vi "SetMenuDisplayed.vi"(8 "error in (no error)":errorcluster, 9 "Displayed":bool, 10 "Tag":string, 11 "Menu in":refnum<class "Menu.lvclass">) -> (0 "error out":errorcluster, 3 "Menu out":refnum<class "Menu.lvclass">)   [LabVIEW 2021, in "Menu.lvlib" / "Menu.lvclass"]
uses:
  Menu.lvclass
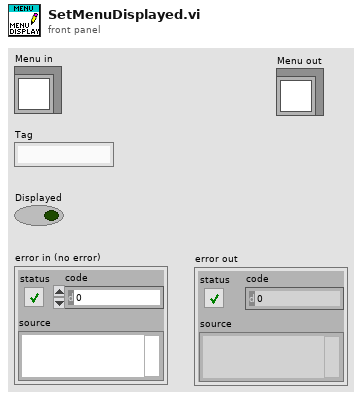
[diagram p1: front panel]
types:
  T1 = typedef "Menu.lvlib/Menu.lvclass/Data.ctl" = cluster{"MenuMap":map{string, T2}, "PictRef":refnum<vi>, "MenuSelectionEvent":refnum<user-event>, "TopMenuSpacing":i32, "MenuSpacing":i32, "CloseEvent":refnum<user-event>, "TR_ManageMenuRef":refnum<vi>, "MenuColors":T4, "RTMPath":path, "RTMVIReference":refnum<vi>, "RTMMenuReference":refnum<k9>, "CtlRef":refnum<vi>, "User-Specified Font":refnum<class "Font.lvclass">, "Desired Font":enum16{"User-specified Font", "Application Font", "System Font", "Dialog Font"}, "SubMenuIcon":T5, "SubMenuIconClosed":refnum<class "Picture2D.lvclass">, "SubMenuIconOpened":refnum<class "Picture2D.lvclass">}
  T2 = typedef "Menu.lvlib/Menu.lvclass/MenuItems.ctl" = cluster{"Item Name":string, "Short Cut":T3, "Checked":bool, "Enable":bool, "After item":string, "Item Tags":string[], "Item Names":string[], "Picture":refnum<class "Image.lvclass">, "Hilite Picture":refnum<class "Image.lvclass">, "Displayed":bool}
  T3 = typedef "LVMenuShortCut.ctl" = cluster{"Include Shift Key?":bool, "Include Ctrl Key?":bool, "Shortcut Key":string}
  T4 = typedef "Menu.lvlib/Menu.lvclass/MenuColors.ctl" = cluster{"Text":refnum<class "Color.lvclass">, "HiliteText":refnum<class "Color.lvclass">, "Background":refnum<class "Color.lvclass">, "BorderColor":refnum<class "Color.lvclass">, "Hilite":refnum<class "Color.lvclass">}
  T5 = typedef "Menu.lvlib/Menu.lvclass/SubMenuIcon.ctl" = enum16{"LabVIEW", "Windows", "Custom"}
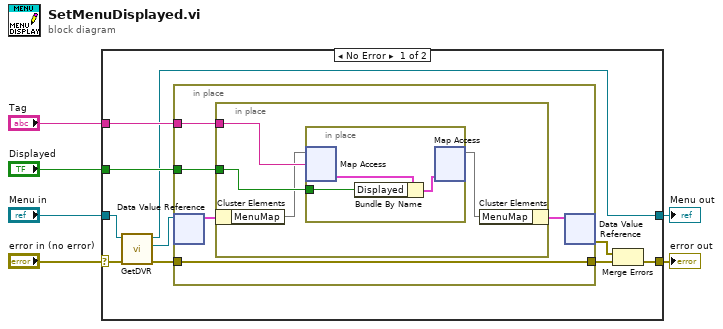
[diagram p0: block diagram]
diagram:
  n1 = case shown="No Error" "error in (no error)" {
    selector: "error in (no error)" -> [w9 w29]
    tunnel: "Tag" -> [w16 _]
    tunnel: "Menu in" -> [w15 w30]
    tunnel: "Displayed" -> [w10 _]
    tunnel: [w7 w30] -> w2
    tunnel: [w8 w29] -> w1
    frame No Error {
      n2 = call "GetDVR.vi"("error in (no error)"=w9, "Menu in"=w15) -> ("error out"=w14:errorcluster, "DVR"=w13:refnum<data-value>, "Menu out"=w7:refnum<class "Menu.lvclass">)  [unwired: 7 in]
      n3 = in-place {
        in-place-border: w14 -> [w21]
        in-place-border: [w21] -> w12
        in-place-border: w16 -> [w20]
        in-place-border: w10 -> [w19]
        n4 = in-place-dvr #1(w13) -> (w18:T1)  [unwired: 1 out]
        n5 = in-place {
          in-place-border: w20 -> [w25]
          in-place-border: w19 -> [w24]
          n6 = in-place-cluster #2(w18) -> ("MenuMap"=w23:map{string, T2})
          n7 = in-place {
            in-place-border: w24 -> [w26]
            n8 = in-place-map #3(w23, w25) -> (w28:T2)  [unwired: 1 in, 1 out]
            n9 = Bundle By Name(cluster=w28, "Displayed"=w26) -> (w27:T2)
            n10 = in-place-map #3(w27) -> (w22:map{string, T2})  [unwired: 1 in, 2 out]
          }
          n11 = in-place-cluster #2("MenuMap"=w22) -> (w17:T1)
        }
        n12 = in-place-dvr #1(w17) -> (w11:errorcluster)  [unwired: 1 out]
      }
      n13 = Merge Errors(w11, w12) -> (w8:errorcluster)
    }
    frame Error {
    }
  }
  "Menu out" <- w2
  "error out" <- w1
